vi "sendPacketsToComponent.vi"(8 "error in (no error)":errorcluster, 11 "TcpServer in":refnum<class "TcpServer.lvclass">) -> (0 "error out":errorcluster, 3 "TcpServer out":refnum<class "TcpServer.lvclass">)   [LabVIEW 2018, in "TcpServer.lvclass"]
doc: "Send TCP packet and connection status to Component."
uses:
  TcpServer.lvclass
  TcpServer.lvclass/TcpServer.ctl
  TcpServerCmd/TcpServerCmd.lvclass/TcpServerCmd.ctl
  TcpServerBase/TcpServerBase.lvclass/TcpServerBase.ctl
  TcpServerCmd/TcpServerCmd.lvclass
  home/pcortes/github/ts_labview_tcp_json/src/TcpServerBase/TcpServerBase.lvclass
  TcpServerBase/TcpServerBase.lvclass
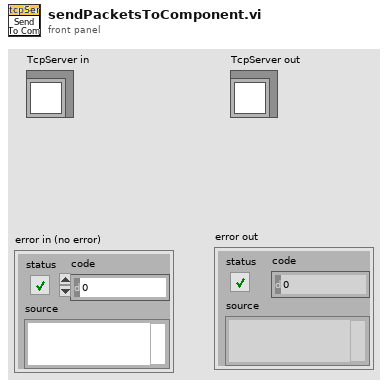
[diagram p1: front panel]
types:
  T1 = typedef "TcpServerCmd.lvclass/userEventTypeDef.ctl" = cluster{"CmdWrite":refnum<user-event>, "EvtWrite":refnum<user-event>, "CmdToServer":refnum<user-event>, "EvtToServer":refnum<user-event>}
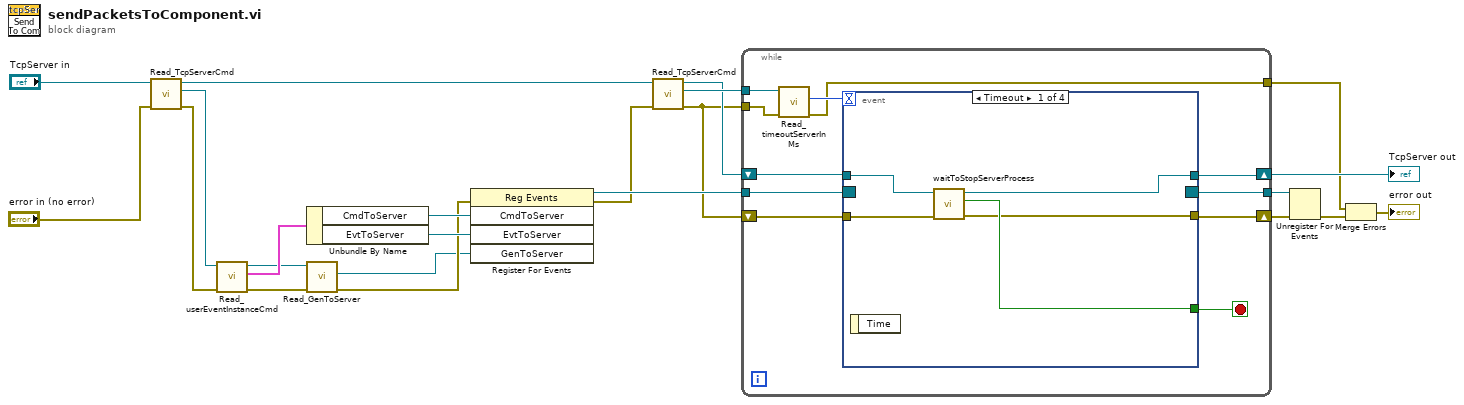
[diagram p0: block diagram]
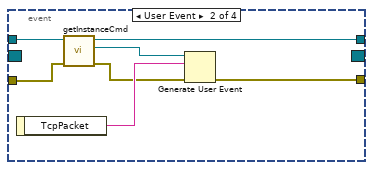
[diagram p2: hidden frame]
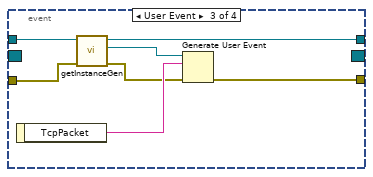
[diagram p3: hidden frame]
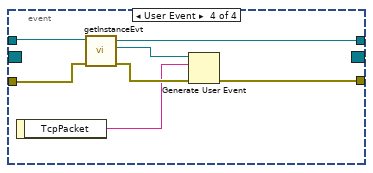
[diagram p4: hidden frame]
diagram:
  n1 = call "Read_TcpServerCmd.vi"("error in (no error)"="error in (no error)", "TcpServer in"="TcpServer in") -> ("error out"=w12:errorcluster, "TcpServerCmd.lvclass"=w6:refnum<class "TcpServerCmd.lvclass">, "TcpServer out"=w19:refnum<class "TcpServer.lvclass">)  [unwired: 7 in]
  n2 = call "Read_userEventInstanceCmd.vi"("error in (no error)"=w12, "TcpServerCmd in"=w6) -> ("error out"=w14:errorcluster, "userEventInstanceCmd"=w18:T1, "TcpServerCmd out"=w15:refnum<class "TcpServerCmd.lvclass">)  [unwired: 7 in]
  n3 = Unbundle By Name(w18) -> ("CmdToServer"=w17:refnum<user-event>, "EvtToServer"=w16:refnum<user-event>)
  n4 = call "Read_GenToServer.vi"("error in (no error)"=w14, "TcpServerBase in"=w15) -> ("error out"=w11:errorcluster, "GenToServer"=w9:refnum<user-event>)  [unwired: 7 in, 1 out]
  n5 = register-events(error in=w11, w17, w16, w9) -> (reference out=w23:refnum<event-registration>, error out=w8:errorcluster)  [unwired: 1 in]
  n6 = call "Read_TcpServerCmd.vi"("error in (no error)"=w8, "TcpServer in"=w19) -> ("error out"=w4:errorcluster, "TcpServerCmd.lvclass"=w7:refnum<class "TcpServerCmd.lvclass">, "TcpServer out"=w5:refnum<class "TcpServer.lvclass">)  [unwired: 7 in]
  n7 = while {
    tunnel: w23 -> [w34]
    tunnel: w7 -> [w32]
    tunnel: [w30] -> w22
    shift-right: [w28] -> w21
    shift-left: w4 -> [w29]
    tunnel: w4 -> [w26]
    shift-right: [w25] -> w3
    shift-left: w5 -> [w27]
    tunnel: [w24] -> w1
    stop <- w31 stop-if-true
    n8 = call "Read_timeoutServerInMs.vi"("error in (no error)"=w26, "TcpServerBase in"=w32) -> ("error out"=w24:errorcluster, "timeoutServerInMs"=w33:i32)  [unwired: 7 in, 1 out]
    n9 = event shown="[0] Timeout" {
      selector: w34 -> [_ _ _ _]
      dyn-events: [_ _ _ _] -> w30
      timeout: w33 -> [_ _ _ _]
      tunnel: [w38 _ _ _] -> w31
      tunnel: w29 -> [w39 w41 w48 w57]
      tunnel: [w37 w43 w50 w55] -> w28
      tunnel: w27 -> [w36 w46 w53 w60]
      tunnel: [w35 w40 w47 w54] -> w25
      event Timeout {
        n10 = event-data() -> ()  [unwired: 1 in, 1 out]
        n11 = call "waitToStopServerProcess.vi"("error in (no error)"=w39, "tcpServer in"=w36) -> ("error out"=w37:errorcluster, "stopProcess"=w38:bool, "tcpServer out"=w35:refnum<class "TcpServer.lvclass">)  [unwired: 6 in, 1 out]
      }
      event User Event {
        n12 = event-data() -> ("TcpPacket"=w44:string)  [unwired: 1 in]
        n13 = call "getInstanceCmd.vi"("error in (no error)"=w41, "tcpServer in"=w46) -> ("error out"=w42:errorcluster, "CmdRead"=w45:refnum<user-event>, "tcpServer out"=w40:refnum<class "TcpServer.lvclass">)  [unwired: 7 in]
        n14 = Generate User Event(user event=w45, event data cluster=w44, error in=w42) -> (error out=w43:errorcluster)  [unwired: 1 in, 1 out]
      }
      event User Event {
        n15 = event-data() -> ("TcpPacket"=w51:string)  [unwired: 1 in]
        n16 = call "getInstanceGen.vi"("error in (no error)"=w48, "tcpServer in"=w53) -> ("error out"=w49:errorcluster, "GenRead"=w52:refnum<user-event>, "tcpServer out"=w47:refnum<class "TcpServer.lvclass">)  [unwired: 7 in]
        n17 = Generate User Event(user event=w52, event data cluster=w51, error in=w49) -> (error out=w50:errorcluster)  [unwired: 1 in, 1 out]
      }
      event User Event {
        n18 = event-data() -> ("TcpPacket"=w56:string)  [unwired: 1 in]
        n19 = call "getInstanceEvt.vi"("error in (no error)"=w57, "tcpServer in"=w60) -> ("error out"=w58:errorcluster, "EvtRead"=w59:refnum<user-event>, "tcpServer out"=w54:refnum<class "TcpServer.lvclass">)  [unwired: 7 in]
        n20 = Generate User Event(user event=w59, event data cluster=w56, error in=w58) -> (error out=w55:errorcluster)  [unwired: 1 in, 1 out]
      }
    }
  }
  "TcpServer out" <- w3
  n21 = Unregister For Events(event registration refnum=w22, error in=w21) -> (error out=w10:errorcluster)
  n22 = Merge Errors(w1, w10) -> (→"error out":errorcluster)
